vi "LSMcontroller_v66_improvedwfhandling.vi"() -> ()   [LabVIEW 2015] (continued)
                            n4742 = call "correctwaveformsizetemp.vi"("new sampling frequency (Hz)"=w1790, "start"=FALSE, "reference waveforms to"=w1802, "Analog waveforms in"=w1800, "stop"=FALSE, "Digital waveforms in"=w1807) -> ("analog wf out"=w1805:waveform(dbl)[], "Digital wf out"=w1803:digitalwaveform[], "measpoints"=w1792:i32)
                            n4743 = local read "wavdet"() -> (w1793:bool)
                            n4744 = local write "Analog Lines Plot"(w1805) -> ()
                            n4745 = call "GetNumCamFramesv2.vi"("Digital Waveform Graph"=w1803) -> ("Numeric"=w1804:i32)  [unwired: 10 in]
                            n4746 = local write "Digital Lines Plot"(w1803) -> ()
                            n4747 = call "waveformsAObuffer.vi"("AO wf in"=w1805, "command"="set") -> ()  [unwired: 1 out]
                            n4748 = call "waveformsDObuffer.vi"("DO wf in"=w1803, "command"="set") -> ()  [unwired: 1 out]
                            n4749 = local write "Total Camera Frames"(w1804) -> ()
                            n4750 = case shown="True" w1793 {
                              tunnel: w1792 -> [_ w1813]
                              frame False {
                              }
                              frame True {
                                n4751 = local write "# of frames"(w1813) -> ()
                              }
                            }
                          }
                        }
                      }
                    }
                  }
                  frame #5 {
                    w1815 = FALSE ("addAO")
                    n4752 = case shown="True" w1814 {
                      frame False {
                      }
                      frame True {
                        n4753 = local write "not loadedml"(FALSE ("not loadedml")) -> ()
                      }
                    }
                    n4754 = local read "finite samples"() -> (w1816:bool)
                    n4755 = local read "continuous"() -> (w1817:bool)
                    n4756 = local read "wavdet"() -> (w1818:bool)
                    n4757 = property on="Load Matlab Waveform" class="Bool (strict)"("Val(Sgnl)"=w1815) -> ()  [unwired: 2 in, 2 out]
                    n4758 = local write "changeAOmatlab"(w1815) -> ()
                    n4759 = call "2pparameters.vi"("command"="get") -> ("params out"=w1821:T10)  [unwired: 1 in]
                    n4760 = Bundle By Name(cluster=w1821, "finite"=w1816, "cont"=w1817, "wavdet"=w1818) -> (w1819:T10)
                    n4761 = call "2pparameters.vi"("Params in"=w1819, "command"="set") -> ()  [unwired: 1 out]
                  }
                }
              }
            }
          }
          event "Load Matlab Waveform DO": Value Change {
            n4762 = event-data() -> ("NewVal"=w1824:bool)  [unwired: 1 in, 5 out]
            n4763 = case shown="True" w1824 {
              frame False {
              }
              frame True {
                n4764 = stacked-sequence {
                  seq-local: [_ _ w1932 _ _] -> [_ _ _ w1947 _]
                  seq-local: [_ _ w1931 _ _] -> [_ _ _ w1946 _]
                  frame #0 {
                    n4765 = local read "Measurement"() -> (w1826:T4)
                    n4766 = case shown="\"X-Y-t movie\", Default" w1826 {
                      frame "X-Y-t movie", Default {
                        n4767 = local read "avpp"() -> (w1847:i32)
                        n4768 = local read "Angle ref"() -> (w1846:dbl)
                        n4769 = local read "ROI Type"() -> (w1845:u16)
                        n4770 = local read "xpixels ref"() -> (w1842:i32)
                        n4771 = local read "Vx-min ref"() -> (w1841:dbl)
                        n4772 = local read "Vx-max ref"() -> (w1840:dbl)
                        n4773 = local read "ypixels ref"() -> (w1838:i32)
                        n4774 = local read "Vy-min ref"() -> (w1839:dbl)
                        n4775 = local read "Vy-max ref"() -> (w1835:dbl)
                        n4776 = local read "Sampling rate"() -> (w1829:dbl)
                        n4777 = local read "finite samples"() -> (w1830:bool)
                        n4778 = local read "continuous"() -> (w1833:bool)
                        n4779 = local read "wavdet"() -> (w1834:bool)
                        n4780 = local read "# of frames"() -> (w1832:i32)
                        n4781 = local read "maxbufferAI"() -> (w1831:i32)
                        n4782 = local read "Override AI buffer"() -> (w1827:bool)
                        n4783 = call "2pparameters.vi"("command"="get") -> ("params out"=w1844:T10)  [unwired: 1 in]
                        n4784 = Bundle By Name(cluster=w1844, "type"="X-Y-t movie", "avpp"=w1847, "Angle Img"=w1846, "Xpixels Img"=w1842, "Vx-min Img"=w1841, "VX-max Img"=w1840, "Ypixels Img"=w1838, "Vy-min Img"=w1839, "Vy-max Img"=w1835, "srate"=w1829, "srate Img"=w1829, "finite"=w1830, "cont"=w1833, "wavdet"=w1834, "measpoints"=w1832, "maxbufferAI"=w1831, "Drawing Mode"=w1845, "Vz-reset"=0.0, "AIoverride"=w1827) -> (w1836:T10)
                        n4785 = call "2pparameters.vi"("Params in"=w1836, "command"="set") -> ()  [unwired: 1 out]
                      }
                      frame "X-Y-Z stack" {
                        n4786 = call "2pparameters.vi"("command"="get") -> ("params out"=w1851:T10)  [unwired: 1 in]
                        n4787 = Bundle By Name(cluster=w1851, "type"="X-Y-Z stack") -> (w1849:T10)
                        n4788 = call "2pparameters.vi"("Params in"=w1849, "command"="set") -> ()  [unwired: 1 out]
                      }
                      frame "Lifetime (scan)" {
                        n4789 = call "2pparameters.vi"("command"="get") -> ("params out"=w1856:T10)  [unwired: 1 in]
                        n4790 = Bundle By Name(cluster=w1856, "type"="Lifetime (scan)") -> (w1854:T10)
                        n4791 = call "2pparameters.vi"("Params in"=w1854, "command"="set") -> ()  [unwired: 1 out]
                      }
                      frame "Lifetime (contour)" {
                        n4792 = local read "Vy-min draw"() -> (w1866:dbl)
                        n4793 = local read "Vy-max draw"() -> (w1865:dbl)
                        n4794 = local read "Vx-min draw"() -> (w1868:dbl)
                        n4795 = local read "Vx-max draw"() -> (w1867:dbl)
                        n4796 = local read "xpixels ref"() -> (w1864:i32)
                        n4797 = local read "ypixels ref"() -> (w1863:i32)
                        n4798 = local read "ROI Type"() -> (w1862:u16)
                        n4799 = local read "srateAODOtt"() -> (w1873:dbl)
                        n4800 = local read "# of frames"() -> (w1878:i32)
                        n4801 = local read "refreshtime"() -> (w1870:dbl)
                        n4802 = local read "Pel"() -> (w1861:dbl)
                        n4803 = local read "bin"() -> (w1876:dbl)
                        n4804 = local read "Override AI buffer"() -> (w1859:bool)
                        n4805 = local read "finite samples"() -> (w1885:bool)
                        n4806 = local read "srateAODOtt"() -> (w1872:dbl)
                        n4807 = local read "srateAODOtt"() -> (w1879:dbl)
                        n4808 = local read "continuous"() -> (w1884:bool)
                        n4809 = local read "Angle ref"() -> (w1869:dbl)
                        n4810 = local read "wavdet"() -> (w1886:bool)
                        n4811 = local read "Vx-ref"() -> (w1881:dbl)
                        n4812 = local read "Vy-ref"() -> (w1883:dbl)
                        n4813 = local read "avpp"() -> (w1882:i32)
                        n4814 = call "tt_timeandsamples.vi"("bin"=w1876, "refreshtime"=w1870, "srateAODOtt"=w1873, "tot#ofsamples"=w1878) -> ("refreshrate"=w1874:dbl, "refreshbuffer"=w1875:i32, "timetracecycles"=w1880:i32)  [unwired: 5 in]
                        n4815 = local read "bin"() -> (w1877:dbl)
                        n4816 = call "2pparameters.vi"("command"="get") -> ("params out"=w1889:T10)  [unwired: 1 in]
                        n4817 = Bundle By Name(cluster=w1889, "Drawing Mode"=w1862, "measpoints"=w1878, "tt_cycles"=w1880, "refreshbuffer"=w1875, "refreshrate"=w1874, "Vx-ref"=w1881, "Vy-ref"=w1883, "srate"=w1872, "finite"=w1885, "cont"=w1884, "wavdet"=w1886, "avpp"=w1882, "srateAODO"=w1879, "bufferAI"=w1875, "bin"=w1877, "Angle Img"=w1869, "Vxminref"=w1868, "Vxmaxref"=w1867, "Vyminref"=w1866, "Vymaxref"=w1865, "Xpixels Img"=w1864, "Ypixels Img"=w1863, "Pel"=w1861, "Vz-reset"=0.0, "AIoverride"=w1859, "type"="Lifetime (contour)") -> (w1887:T10)
                        n4818 = Reciprocal(x=w1874) -> (1/x=w1871:dbl)
                        n4819 = local write "refreshtime"(w1871) -> ()
                        n4820 = call "2pparameters.vi"("Params in"=w1887, "command"="set") -> ()  [unwired: 1 out]
                      }
                      frame "X-Y-Z-t movie" {
                      }
                      frame "linescan" {
                      }
                      frame "Timetrace" {
                        n4821 = local read "Vy-min draw"() -> (w1899:dbl)
                        n4822 = local read "Vy-max draw"() -> (w1898:dbl)
                        n4823 = local read "Vx-min draw"() -> (w1901:dbl)
                        n4824 = local read "Vx-max draw"() -> (w1900:dbl)
                        n4825 = local read "xpixels ref"() -> (w1897:i32)
                        n4826 = local read "ypixels ref"() -> (w1896:i32)
                        n4827 = local read "ROI Type"() -> (w1895:u16)
                        n4828 = local read "srateAODOtt"() -> (w1906:dbl)
                        n4829 = local read "# of frames"() -> (w1911:i32)
                        n4830 = local read "refreshtime"() -> (w1903:dbl)
                        n4831 = local read "Pel"() -> (w1894:dbl)
                        n4832 = local read "bin"() -> (w1909:dbl)
                        n4833 = local read "Override AI buffer"() -> (w1892:bool)
                        n4834 = local read "finite samples"() -> (w1918:bool)
                        n4835 = local read "srateAODOtt"() -> (w1905:dbl)
                        n4836 = local read "srateAODOtt"() -> (w1912:dbl)
                        n4837 = local read "continuous"() -> (w1917:bool)
                        n4838 = local read "Angle ref"() -> (w1902:dbl)
                        n4839 = local read "wavdet"() -> (w1919:bool)
                        n4840 = local read "Vx-ref"() -> (w1914:dbl)
                        n4841 = local read "Vy-ref"() -> (w1916:dbl)
                        n4842 = local read "avpp"() -> (w1915:i32)
                        n4843 = call "tt_timeandsamples.vi"("bin"=w1909, "refreshtime"=w1903, "srateAODOtt"=w1906, "tot#ofsamples"=w1911) -> ("refreshrate"=w1907:dbl, "refreshbuffer"=w1908:i32, "timetracecycles"=w1913:i32)  [unwired: 5 in]
                        n4844 = local read "bin"() -> (w1910:dbl)
                        n4845 = call "2pparameters.vi"("command"="get") -> ("params out"=w1922:T10)  [unwired: 1 in]
                        n4846 = Bundle By Name(cluster=w1922, "Drawing Mode"=w1895, "measpoints"=w1911, "tt_cycles"=w1913, "refreshbuffer"=w1908, "refreshrate"=w1907, "Vx-ref"=w1914, "Vy-ref"=w1916, "srate"=w1905, "finite"=w1918, "cont"=w1917, "wavdet"=w1919, "avpp"=w1915, "srateAODO"=w1912, "bufferAI"=w1908, "bin"=w1910, "Angle Img"=w1902, "Vxminref"=w1901, "Vxmaxref"=w1900, "Vyminref"=w1899, "Vymaxref"=w1898, "Xpixels Img"=w1897, "Ypixels Img"=w1896, "Pel"=w1894, "Vz-reset"=0.0, "AIoverride"=w1892, "type"="Timetrace") -> (w1920:T10)
                        n4847 = Reciprocal(x=w1907) -> (1/x=w1904:dbl)
                        n4848 = local write "refreshtime"(w1904) -> ()
                        n4849 = call "2pparameters.vi"("Params in"=w1920, "command"="set") -> ()  [unwired: 1 out]
                      }
                      frame "Lifetime (point)" {
                      }
                    }
                    n4850 = local write "changeDOmatlab"(TRUE ("addAO")) -> ()
                  }
                  frame #1 {
                    w1925 = FALSE ("wavdet")
                    n4851 = call "2pparameters.vi"("command"="get") -> ("params out"=w1929:T10)  [unwired: 1 in]
                    n4852 = Bundle By Name(cluster=w1929, "finite"=w1925, "cont"=w1925, "wavdet"=TRUE) -> (w1926:T10)
                    n4853 = call "2pparameters.vi"("Params in"=w1926, "command"="set") -> ()  [unwired: 1 out]
                  }
                  frame #2 {
                    n4854 = local read "DO channels"() -> (w1934:u16)
                    n4855 = call "2pparameters.vi"("command"="get") -> ("params out"=w1936:T10)  [unwired: 1 in]
                    n4856 = Unbundle By Name(w1936) -> ("aDO"=w1935:u32[])
                    n4857 = Search 1D Array(1D array=w1935, element=w1934) -> (index of element=w1932:i32)  [unwired: 1 in]
                    n4858 = Greater?(x=w1932, y=-1) -> (0:w1931:bool)
                    n4859 = case shown="True" w1931 {
                      tunnel: w1932 -> [_ w1943]
                      frame False {
                      }
                      frame True {
                        n4860 = local read "Meastab"() -> (w1939:enum32{"X-Y Image", "Linescan", "Timetrace"})
                        n4861 = local read "Matlab waveform path DO"() -> (w1941:path)
                        n4862 = local read "Matlab padding value DO"() -> (w1942:dbl)
                        n4863 = case shown="\"Timetrace\"" w1939 {
                          tunnel: [w1944 w1945] -> w1938
                          frame "X-Y Image", Default {
                            n4864 = local read "Sampling rate"() -> (w1944:dbl)
                          }
                          frame "Timetrace" {
                            n4865 = local read "srateAODOtt"() -> (w1945:dbl)
                          }
                        }
                        n4866 = call "matlabwfexistsdialogue.vi"("Matlab waveform path"=w1941) -> ("mtalab waveform path out"=w1940:path)
                        n4867 = call "replace DO matlab param.vi"("Sampling frequency (Hz)"=w1938, "matlab wave number"=w1940, "index of DO wave"=w1943, "padding value"=w1942) -> ()  [unwired: 7 in]
                      }
                    }
                  }
                  frame #3 {
                    n4868 = case shown="True" w1946 {
                      tunnel: w1947 -> [_ w1956]
                      frame False {
                      }
                      frame True {
                        n4869 = local read "Meastab"() -> (w1951:enum32{"X-Y Image", "Linescan", "Timetrace"})
                        n4870 = call "waveformparamsv2.vi"("command"="get") -> ("Params out"=w1969:T14)  [unwired: 4 in, 2 out]
                        n4871 = Unbundle By Name(w1969) -> ("DO parameters"=w1968:T17)
                        n4872 = case shown="\"Timetrace\"" w1951 {
                          tunnel: [w1971 w1972] -> w1950
                          frame "X-Y Image", Default {
                            n4873 = local read "Sampling rate"() -> (w1971:dbl)
                          }
                          frame "Timetrace" {
                            n4874 = local read "srateAODOtt"() -> (w1972:dbl)
                          }
                        }
                        n4875 = Index Array(array=w1968, index=w1956) -> (element=w1955:T18)
                        n4876 = call "waveformsDObuffer.vi"("command"="get") -> ("DO wf out"=w1966:digitalwaveform[])  [unwired: 1 in]
                        n4877 = property on="refwf" class="Ring (strict)"() -> ("RingText.Text"=w1958:string)  [unwired: 2 in, 2 out]
                        n4878 = call "matlabDOwffromparam.vi"("waveform params"=w1955) -> ("digital waveform"=w1954:digitalwaveform)
                        n4879 = Replace Array Subset(array=w1966, new element=w1954, index=w1956) -> (w1957:digitalwaveform[])
                        n4880 = call "waveformsAObuffer.vi"("command"="get") -> ("AO wf out"=w1965:waveform(dbl)[])  [unwired: 1 in]
                        n4881 = local read "wavdet"() -> (w1953:bool)
                        n4882 = call "correctwaveformsizetemp.vi"("new sampling frequency (Hz)"=w1950, "start"=FALSE, "reference waveforms to"=w1958, "Analog waveforms in"=w1965, "stop"=FALSE, "Digital waveforms in"=w1957) -> ("analog wf out"=w1961:waveform(dbl)[], "Digital wf out"=w1959:digitalwaveform[], "measpoints"=w1952:i32)
                        n4883 = local write "Analog Lines Plot"(w1961) -> ()
                        n4884 = call "GetNumCamFramesv2.vi"("Digital Waveform Graph"=w1959) -> ("Numeric"=w1960:i32)  [unwired: 10 in]
                        n4885 = local write "Digital Lines Plot"(w1959) -> ()
                        n4886 = case shown="True" w1953 {
                          tunnel: w1952 -> [_ w1973]
                          frame False {
                          }
                          frame True {
                            n4887 = local write "# of frames"(w1973) -> ()
                          }
                        }
                        n4888 = call "waveformsAObuffer.vi"("AO wf in"=w1961, "command"="set") -> ()  [unwired: 1 out]
                        n4889 = call "waveformsDObuffer.vi"("DO wf in"=w1959, "command"="set") -> ()  [unwired: 1 out]
                        n4890 = local write "Total Camera Frames"(w1960) -> ()
                      }
                    }
                  }
                  frame #4 {
                    w1975 = FALSE ("addAO")
                    n4891 = local read "finite samples"() -> (w1976:bool)
                    n4892 = local read "continuous"() -> (w1977:bool)
                    n4893 = local read "wavdet"() -> (w1978:bool)
                    n4894 = call "2pparameters.vi"("command"="get") -> ("params out"=w1981:T10)  [unwired: 1 in]
                    n4895 = Bundle By Name(cluster=w1981, "finite"=w1976, "cont"=w1977, "wavdet"=w1978) -> (w1979:T10)
                    n4896 = local write "not loadedDOml"(FALSE ("not loadedDO")) -> ()
                    n4897 = local write "changeDOmatlab"(w1975) -> ()
                    n4898 = property on="Load Matlab Waveform DO" class="Bool (strict)"("Val(Sgnl)"=w1975) -> ()  [unwired: 2 in, 2 out]
                    n4899 = call "2pparameters.vi"("Params in"=w1979, "command"="set") -> ()  [unwired: 1 out]
                  }
                }
              }
            }
          }
          event "Add settings": Value Change {
            n4900 = event-data() -> ("NewVal"=w1983:bool)  [unwired: 1 in, 5 out]
            n4901 = case shown="True" w1983 {
              frame False {
              }
              frame True {
                n4902 = stacked-sequence {
                  frame #0 {
                    n4903 = call "wfsettings.vi"("command"="get") -> ("wfsettings out"=w1986:T27)  [unwired: 2 in, 1 out]
                    n4904 = in-place {
                      n4905 = in-place-cluster #53(w1986) -> ("settings names"=w1991:string[], "settings locations"=w1993:path[])
                      n4906 = local read "Setting location"() -> (w1989:path)
                      n4907 = local read "Nickname"() -> (w1988:string)
                      n4908 = Build Array (concatenate)(w1991, w1988) -> (w1990:string[])
                      n4909 = property on="Loaded settings" class="Ring (strict)"("Strings []"=w1990) -> ()  [unwired: 2 in, 2 out]
                      n4910 = Build Array (concatenate)(w1993, w1989) -> (w1992:path[])
                      n4911 = in-place-cluster #53("settings names"=w1990, "settings locations"=w1992) -> (w1984:T27)
                    }
                    n4912 = call "wfsettings.vi"("wfsettings in"=w1984, "command"="set") -> ()  [unwired: 1 in, 2 out]
                  }
                  frame #1 {
                    n4913 = property on="Add settings" class="Bool (strict)"("Val(Sgnl)"=FALSE ("Value (Signaling)")) -> ()  [unwired: 2 in, 2 out]
                  }
                }
              }
            }
          }
          event "Rem setting": Value Change {
            n4914 = event-data() -> ("NewVal"=w1995:bool)  [unwired: 1 in, 5 out]
            n4915 = case shown="True" w1995 {
              frame False {
              }
              frame True {
                n4916 = stacked-sequence {
                  frame #0 {
                    n4917 = call "wfsettings.vi"("command"="get") -> ("wfsettings out"=w1998:T27)  [unwired: 2 in, 1 out]
                    n4918 = in-place {
                      n4919 = in-place-cluster #54(w1998) -> ("settings names"=w2003:string[], "settings locations"=w2001:path[])
                      n4920 = property on="Loaded settings" class="Ring (strict)"() -> ("RingText.Text"=w2004:string)  [unwired: 2 in, 2 out]
                      n4921 = Search 1D Array(1D array=w2003, element=w2004) -> (index of element=w2005:i32)  [unwired: 1 in]
                      n4922 = Delete From Array(array=w2003, index=w2005) -> (array with subset deleted=w2002:string[])  [unwired: 1 in, 1 out]
                      n4923 = Delete From Array(array=w2001, index=w2005) -> (array with subset deleted=w2000:path[])  [unwired: 1 in, 1 out]
                      n4924 = property on="Loaded settings" class="Ring (strict)"("Strings []"=w2002) -> ()  [unwired: 2 in, 2 out]
                      n4925 = in-place-cluster #54("settings names"=w2002, "settings locations"=w2000) -> (w1996:T27)
                    }
                    n4926 = call "wfsettings.vi"("wfsettings in"=w1996, "command"="set") -> ()  [unwired: 1 in, 2 out]
                  }
                  frame #1 {
                    n4927 = property on="Rem setting" class="Bool (strict)"("Val(Sgnl)"=FALSE ("Value (Signaling)")) -> ()  [unwired: 2 in, 2 out]
                  }
                }
              }
            }
          }
          event "Update settings": Value Change {
            n4928 = event-data() -> ("NewVal"=w2007:bool)  [unwired: 1 in, 5 out]
            n4929 = case shown="True" w2007 {
              frame False {
              }
              frame True {
                n4930 = stacked-sequence {
                  frame #0 {
                    n4931 = local read "Measurement"() -> (w2008:T4)
                    n4932 = case shown="\"Timetrace\"" w2008 {
                      frame "X-Y-t movie", Default {
                        n4933 = local read "avpp"() -> (w2029:i32)
                        n4934 = local read "Angle ref"() -> (w2028:dbl)
                        n4935 = local read "ROI Type"() -> (w2027:u16)
                        n4936 = local read "xpixels ref"() -> (w2024:i32)
                        n4937 = local read "Vx-min ref"() -> (w2023:dbl)
                        n4938 = local read "Vx-max ref"() -> (w2022:dbl)
                        n4939 = local read "ypixels ref"() -> (w2020:i32)
                        n4940 = local read "Vy-min ref"() -> (w2021:dbl)
                        n4941 = local read "Vy-max ref"() -> (w2017:dbl)
                        n4942 = local read "Sampling rate"() -> (w2011:dbl)
                        n4943 = local read "finite samples"() -> (w2012:bool)
                        n4944 = local read "continuous"() -> (w2015:bool)
                        n4945 = local read "wavdet"() -> (w2016:bool)
                        n4946 = local read "# of frames"() -> (w2014:i32)
                        n4947 = local read "maxbufferAI"() -> (w2013:i32)
                        n4948 = local read "Override AI buffer"() -> (w2009:bool)
                        n4949 = call "2pparameters.vi"("command"="get") -> ("params out"=w2026:T10)  [unwired: 1 in]
                        n4950 = Bundle By Name(cluster=w2026, "type"="X-Y-t movie", "avpp"=w2029, "Angle Img"=w2028, "Xpixels Img"=w2024, "Vx-min Img"=w2023, "VX-max Img"=w2022, "Ypixels Img"=w2020, "Vy-min Img"=w2021, "Vy-max Img"=w2017, "srate"=w2011, "srate Img"=w2011, "finite"=w2012, "cont"=w2015, "wavdet"=w2016, "measpoints"=w2014, "maxbufferAI"=w2013, "Drawing Mode"=w2027, "Vz-reset"=0.0, "AIoverride"=w2009) -> (w2018:T10)
                        n4951 = call "2pparameters.vi"("Params in"=w2018, "command"="set") -> ()  [unwired: 1 out]
                      }
                      frame "X-Y-Z stack" {
                        n4952 = call "2pparameters.vi"("command"="get") -> ("params out"=w2033:T10)  [unwired: 1 in]
                        n4953 = Bundle By Name(cluster=w2033, "type"="X-Y-Z stack") -> (w2031:T10)
                        n4954 = call "2pparameters.vi"("Params in"=w2031, "command"="set") -> ()  [unwired: 1 out]
                      }
                      frame "Lifetime (scan)" {
                        n4955 = call "2pparameters.vi"("command"="get") -> ("params out"=w2038:T10)  [unwired: 1 in]
                        n4956 = Bundle By Name(cluster=w2038, "type"="Lifetime (scan)") -> (w2036:T10)
                        n4957 = call "2pparameters.vi"("Params in"=w2036, "command"="set") -> ()  [unwired: 1 out]
                      }
                      frame "Lifetime (contour)" {
                        n4958 = local read "Vy-min draw"() -> (w2048:dbl)
                        n4959 = local read "Vy-max draw"() -> (w2047:dbl)
                        n4960 = local read "Vx-min draw"() -> (w2050:dbl)
                        n4961 = local read "Vx-max draw"() -> (w2049:dbl)
                        n4962 = local read "xpixels ref"() -> (w2046:i32)
                        n4963 = local read "ypixels ref"() -> (w2045:i32)
                        n4964 = local read "ROI Type"() -> (w2044:u16)
                        n4965 = local read "srateAODOtt"() -> (w2055:dbl)
                        n4966 = local read "# of frames"() -> (w2060:i32)
                        n4967 = local read "refreshtime"() -> (w2052:dbl)
                        n4968 = local read "Pel"() -> (w2043:dbl)
                        n4969 = local read "bin"() -> (w2058:dbl)
                        n4970 = local read "Override AI buffer"() -> (w2041:bool)
                        n4971 = local read "finite samples"() -> (w2067:bool)
                        n4972 = local read "srateAODOtt"() -> (w2054:dbl)
                        n4973 = local read "srateAODOtt"() -> (w2061:dbl)
                        n4974 = local read "continuous"() -> (w2066:bool)
                        n4975 = local read "Angle ref"() -> (w2051:dbl)
                        n4976 = local read "wavdet"() -> (w2068:bool)
                        n4977 = local read "Vx-ref"() -> (w2063:dbl)
                        n4978 = local read "Vy-ref"() -> (w2065:dbl)
                        n4979 = local read "avpp"() -> (w2064:i32)
                        n4980 = call "tt_timeandsamples.vi"("bin"=w2058, "refreshtime"=w2052, "srateAODOtt"=w2055, "tot#ofsamples"=w2060) -> ("refreshrate"=w2056:dbl, "refreshbuffer"=w2057:i32, "timetracecycles"=w2062:i32)  [unwired: 5 in]
                        n4981 = local read "bin"() -> (w2059:dbl)
                        n4982 = call "2pparameters.vi"("command"="get") -> ("params out"=w2071:T10)  [unwired: 1 in]
                        n4983 = Bundle By Name(cluster=w2071, "Drawing Mode"=w2044, "measpoints"=w2060, "tt_cycles"=w2062, "refreshbuffer"=w2057, "refreshrate"=w2056, "Vx-ref"=w2063, "Vy-ref"=w2065, "srate"=w2054, "finite"=w2067, "cont"=w2066, "wavdet"=w2068, "avpp"=w2064, "srateAODO"=w2061, "bufferAI"=w2057, "bin"=w2059, "Angle Img"=w2051, "Vxminref"=w2050, "Vxmaxref"=w2049, "Vyminref"=w2048, "Vymaxref"=w2047, "Xpixels Img"=w2046, "Ypixels Img"=w2045, "Pel"=w2043, "Vz-reset"=0.0, "AIoverride"=w2041, "type"="Lifetime (contour)") -> (w2069:T10)
                        n4984 = Reciprocal(x=w2056) -> (1/x=w2053:dbl)
                        n4985 = local write "refreshtime"(w2053) -> ()
                        n4986 = call "2pparameters.vi"("Params in"=w2069, "command"="set") -> ()  [unwired: 1 out]
                      }
                      frame "X-Y-Z-t movie" {
                      }
                      frame "linescan" {
                      }
                      frame "Timetrace" {
                        n4987 = local read "Vy-min draw"() -> (w2081:dbl)
                        n4988 = local read "Vy-max draw"() -> (w2080:dbl)
                        n4989 = local read "Vx-min draw"() -> (w2083:dbl)
                        n4990 = local read "Vx-max draw"() -> (w2082:dbl)
                        n4991 = local read "xpixels ref"() -> (w2079:i32)
                        n4992 = local read "ypixels ref"() -> (w2078:i32)
                        n4993 = local read "ROI Type"() -> (w2077:u16)
                        n4994 = local read "srateAODOtt"() -> (w2088:dbl)
                        n4995 = local read "# of frames"() -> (w2093:i32)
                        n4996 = local read "refreshtime"() -> (w2085:dbl)
                        n4997 = local read "Pel"() -> (w2076:dbl)
                        n4998 = local read "bin"() -> (w2091:dbl)
                        n4999 = local read "Override AI buffer"() -> (w2074:bool)
                        n5000 = local read "finite samples"() -> (w2100:bool)
                        n5001 = local read "srateAODOtt"() -> (w2087:dbl)
                        n5002 = local read "srateAODOtt"() -> (w2094:dbl)
                        n5003 = local read "continuous"() -> (w2099:bool)
                        n5004 = local read "Angle ref"() -> (w2084:dbl)
                        n5005 = local read "wavdet"() -> (w2101:bool)
                        n5006 = local read "Vx-ref"() -> (w2096:dbl)
                        n5007 = local read "Vy-ref"() -> (w2098:dbl)
                        n5008 = local read "avpp"() -> (w2097:i32)
                        n5009 = call "tt_timeandsamples.vi"("bin"=w2091, "refreshtime"=w2085, "srateAODOtt"=w2088, "tot#ofsamples"=w2093) -> ("refreshrate"=w2089:dbl, "refreshbuffer"=w2090:i32, "timetracecycles"=w2095:i32)  [unwired: 5 in]
                        n5010 = local read "bin"() -> (w2092:dbl)
                        n5011 = call "2pparameters.vi"("command"="get") -> ("params out"=w2104:T10)  [unwired: 1 in]
                        n5012 = Bundle By Name(cluster=w2104, "Drawing Mode"=w2077, "measpoints"=w2093, "tt_cycles"=w2095, "refreshbuffer"=w2090, "refreshrate"=w2089, "Vx-ref"=w2096, "Vy-ref"=w2098, "srate"=w2087, "finite"=w2100, "cont"=w2099, "wavdet"=w2101, "avpp"=w2097, "srateAODO"=w2094, "bufferAI"=w2090, "bin"=w2092, "Angle Img"=w2084, "Vxminref"=w2083, "Vxmaxref"=w2082, "Vyminref"=w2081, "Vymaxref"=w2080, "Xpixels Img"=w2079, "Ypixels Img"=w2078, "Pel"=w2076, "Vz-reset"=0.0, "AIoverride"=w2074, "type"="Timetrace") -> (w2102:T10)
                        n5013 = Reciprocal(x=w2089) -> (1/x=w2086:dbl)
                        n5014 = local write "refreshtime"(w2086) -> ()
                        n5015 = call "2pparameters.vi"("Params in"=w2102, "command"="set") -> ()  [unwired: 1 out]
                      }
                      frame "Lifetime (point)" {
                      }
                    }
                  }
                  frame #1 {
                    w2107 = FALSE ("wavdet")
                    n5016 = call "2pparameters.vi"("command"="get") -> ("params out"=w2111:T10)  [unwired: 1 in]
                    n5017 = Bundle By Name(cluster=w2111, "finite"=w2107, "cont"=w2107, "wavdet"=TRUE) -> (w2108:T10)
                    n5018 = call "2pparameters.vi"("Params in"=w2108, "command"="set") -> ()  [unwired: 1 out]
                  }
                  frame #2 {
                    n5019 = property on="Loaded settings" class="Ring (strict)"() -> ("RingText.Text"=w2113:string)  [unwired: 2 in, 2 out]
                    n5020 = control-ref of="Analog Lines Plot"() -> (w2115:refnum<vi>)
                    n5021 = control-ref of="Digital Lines Plot"() -> (w2114:refnum<vi>)
                    n5022 = call "Usedlinesfromsettingsfile.vi"("sertting"=w2113) -> ("used AO names"=w2119:string[], "used AO lines"=w2118:tag[], "used DO names"=w2117:string[], "used DO lines"=w2116:tag[])
                    n5023 = call "loadAODOwfparamsfromsettingsfile.vi"("sertting"=w2113) -> ()
                    n5024 = call "prepAOWaveplot.vi"("WaveformGraph in"=w2115, "Analog Used Names"=w2119) -> ()  [unwired: 1 in]
                    n5025 = local write "Analog Used Names"(w2119) -> ()
                    n5026 = local write "Analog Used Lines"(w2118) -> ()
                    n5027 = call "prepDOWaveplot.vi"("DigitalGraph in"=w2114, "used DO names"=w2117) -> ()  [unwired: 1 in]
                    n5028 = local write "Digital Used Names"(w2117) -> ()
                    n5029 = local write "Digital Used Lines"(w2116) -> ()
                  }
                  frame #3 {
                    n5030 = call "waveformparamsv2.vi"("command"="get") -> ("Params out"=w2136:T14)  [unwired: 4 in, 2 out]
                    n5031 = Unbundle By Name(w2136) -> ("AO parameters"=w2137:T15, "DO parameters"=w2138:T17)
                    n5032 = for {
                      tunnel: w2137 -> [w2158] mode=indexing
                      tunnel: [w2156] -> w2139 mode=indexing
                      tunnel: [w2155] -> w2124 mode=indexing
                      tunnel: [w2153] -> w2127 mode=indexing
                      i -> [w2157]
                      n5033 = Unbundle By Name(w2158) -> ("AOtab"=w2159:dbl)
                      n5034 = To Long Integer(number=w2159) -> (32bit integer=w2152:i32)
                      n5035 = case shown="2" w2152 {
                        tunnel: w2158 -> [_ w2170 w2172 w2174]
                        tunnel: [_ w2169 w2171 w2173] -> w2154
                        frame -1 {
                        }
                        frame 0, Default {
                          n5036 = call "generateRampedSquareWave_fromAOparameters.vi"("AO params"=w2170) -> ("Waveform"=w2169:waveform(dbl))  [unwired: 1 out]
                        }
                        frame 1 {
                          n5037 = call "generateTriWave_fromAOparameters.vi"("AO params"=w2172) -> ("Waveform"=w2171:waveform(dbl))  [unwired: 1 out]
                        }
                        frame 2 {
                          n5038 = call "matlabAOwffromparam.vi"("Cluster"=w2174) -> ("Waveform"=w2173:waveform(dbl))  [unwired: 1 out]
                        }
                      }
                      n5039 = case shown="0" w2157 {
                        tunnel: [w2164 -1] -> w2156
                        tunnel: [w2163 w2167] -> w2155
                        tunnel: w2154 -> [w2163 w2167]
                        tunnel: [w2160 -1.0] -> w2153
                        frame 0 {
                          n5040 = Unbundle By Name(w2163) -> ("dt"=w2162:dbl, "Y"=w2165:dbl[])
                          n5041 = Reciprocal(x=w2162) -> (1/x=w2161:dbl)
                          n5042 = Array Size(array=w2165) -> (size(s)=w2164:i32)
                          n5043 = Round To Nearest(number=w2161) -> (nearest integer value=w2160:dbl)
                        }
                        frame 1, Default {
                        }
                      }
                    }
                    n5044 = Index Array(array=w2139, index=0) -> (element=w2141:i32)
                    n5045 = Index Array(array=w2127, index=0) -> (element=w2126:dbl)
                    n5046 = for {
                      tunnel: w2138 -> [w2146] mode=indexing
                      tunnel: [w2144] -> w2125 mode=indexing
                      tunnel: w2141 -> [w2143]
                      n5047 = Unbundle By Name(w2146) -> ("DOtab"=w2145:dbl)
                      n5048 = case shown="0, Default" w2145 {
                        tunnel: w2146 -> [w2149 w2151]
                        tunnel: w2143 -> [w2148 _]
                        tunnel: [w2147 w2150] -> w2144
                        frame 0, Default {
                          n5049 = call "simple digital from wf params.vi"("waveform params"=w2149, "number of samples"=w2148) -> ("digital waveform"=w2147:digitalwaveform)
                        }
                        frame 1 {
                          n5050 = call "matlabDOwffromparam.vi"("waveform params"=w2151) -> ("digital waveform"=w2150:digitalwaveform)
                        }
                      }
                    }
                    n5051 = property on="refwf" class="Ring (strict)"() -> ("RingText.Text"=w2129:string)  [unwired: 2 in, 2 out]
                    n5052 = call "correctwaveformsizetemp.vi"("new sampling frequency (Hz)"=w2126, "start"=FALSE, "reference waveforms to"=w2129, "Analog waveforms in"=w2124, "stop"=FALSE, "Digital waveforms in"=w2125) -> ("analog wf out"=w2123:waveform(dbl)[], "Digital wf out"=w2122:digitalwaveform[], "measpoints"=w2120:i32)
                    n5053 = local read "wavdet"() -> (w2121:bool)
                    n5054 = case shown="True" w2121 {
                      tunnel: w2120 -> [_ w2142]
                      frame False {
                      }
                      frame True {
                        n5055 = local write "# of frames"(w2142) -> ()
                      }
                    }
                    n5056 = local write "Analog Lines Plot"(w2123) -> ()
                    n5057 = local write "Digital Lines Plot"(w2122) -> ()
                    n5058 = call "GetNumCamFramesv2.vi"("Digital Waveform Graph"=w2122) -> ("Numeric"=w2134:i32)  [unwired: 10 in]
                    n5059 = call "waveformsAObuffer.vi"("AO wf in"=w2123, "command"="set") -> ()  [unwired: 1 out]
                    n5060 = call "waveformsDObuffer.vi"("DO wf in"=w2122, "command"="set") -> ()  [unwired: 1 out]
                    n5061 = local write "Total Camera Frames"(w2134) -> ()
                  }
                  frame #4 {
                    n5062 = local read "AO channels"() -> (w2175:u32)
                    n5063 = call "2pparameters.vi"("command"="get") -> ("params out"=w2177:T10)  [unwired: 1 in]
                    n5064 = Unbundle By Name(w2177) -> ("aAO"=w2176:u32[])
                    n5065 = Search 1D Array(1D array=w2176, element=w2175) -> (index of element=w2179:i32)  [unwired: 1 in]
                    n5066 = Equal?(x=w2179, y=-1.0) -> (x = y?=w2180:bool)
                    n5067 = case shown="False" w2180 {
                      tunnel: w2179 -> [w2205 _]
                      frame False {
                        n5068 = call "waveformparamsv2.vi"("command"="get") -> ("Params out"=w2188:T14)  [unwired: 4 in, 2 out]
                        n5069 = Unbundle By Name(w2188) -> ("AO parameters"=w2187:T15)
                        n5070 = Index Array(array=w2187, index=w2205) -> (element=w2204:T16)
                        n5071 = Unbundle By Name(w2204) -> ("AOtab"=w2185:dbl, "Repeats"=w2203:dbl, "Cycles"=w2202:dbl, "Start amplitude (V)"=w2201:dbl, "Baseline (V)"=w2200:dbl, "Step size (V)"=w2199:dbl, "DC (%)"=w2198:dbl, "Sampling frequency (Hz)"=w2197:dbl, "Period (ms)"=w2196:dbl, "Offset (V)"=w2195:dbl, "Amplitude (V)"=w2194:dbl, "Frequency"=w2193:dbl, "Tri Repeats"=w2192:dbl, "phase shift (ms)"=w2191:dbl, "Pulses"=w2190:dbl, "Tri phase"=w2186:dbl, "padding value"=w2182:dbl, "Matlab wave file"=w2183:path)
                        n5072 = To Unsigned Long Integer(number=w2185) -> (unsigned 32bit integer=w2184:u32)
                        n5073 = local write "Build analog waveform tabs"(w2184) -> ()
                        n5074 = local write "Matlab waveform path"(w2183) -> ()
                        n5075 = local write "phase shift (ms)"(w2191) -> ()
                        n5076 = local write "Repeats"(w2203) -> ()
                        n5077 = local write "Cycles"(w2202) -> ()
                        n5078 = local write "Amplitude (V)"(w2194) -> ()
                        n5079 = local write "Matlab padding value"(w2182) -> ()
                        n5080 = local write "Tri padding value"(w2182) -> ()
                        n5081 = local write "Start amplitude (V)"(w2201) -> ()
                        n5082 = local write "Tri Phase (s)"(w2186) -> ()
                        n5083 = local write "Period (ms)"(w2196) -> ()
                        n5084 = local write "Tri Repeats"(w2192) -> ()
                        n5085 = local write "Offset (V)"(w2195) -> ()
                        n5086 = local write "Frequency"(w2193) -> ()
                        n5087 = local write "Pulses"(w2190) -> ()
                        n5088 = local write "padding value"(w2182) -> ()
                        n5089 = local write "Sampling rate \ncurrent wf"(w2197) -> ()
                        n5090 = local write "Baseline (V)"(w2200) -> ()
                        n5091 = local write "Step size (V)"(w2199) -> ()
                        n5092 = local write "DC (%)"(w2198) -> ()
                      }
                      frame True {
                      }
                    }
                  }
                  frame #5 {
                    n5093 = local read "DO channels"() -> (w2208:u16)
                    n5094 = call "2pparameters.vi"("command"="get") -> ("params out"=w2210:T10)  [unwired: 1 in]
                    n5095 = Unbundle By Name(w2210) -> ("aDO"=w2209:u32[])
                    n5096 = Search 1D Array(1D array=w2209, element=w2208) -> (index of element=w2207:i32)  [unwired: 1 in]
                    n5097 = Equal?(x=w2207, y=-1.0) -> (x = y?=w2206:bool)
                    n5098 = case shown="False" w2206 {
                      tunnel: w2207 -> [w2225 _]
                      frame False {
                        n5099 = call "waveformparamsv2.vi"("command"="get") -> ("Params out"=w2219:T14)  [unwired: 4 in, 2 out]
                        n5100 = Unbundle By Name(w2219) -> ("DO parameters"=w2217:T17)
                        n5101 = Index Array(array=w2217, index=w2225) -> (element=w2224:T18)
                        n5102 = Unbundle By Name(w2224) -> ("Digital DC (%)"=w2223:dbl, "Digital phase"=w2222:dbl, "Digital Freq (Hz)"=w2221:dbl, "Sampling frequency (Hz)"=w2220:dbl, "Digital time offset (s)"=w2216:dbl, "padding value"=w2215:dbl, "matlab wave file"=w2214:path, "DOtab"=w2213:dbl)
                        n5103 = local write "Build digital waveform tabs"(w2213) -> ()
                        n5104 = local write "Digital DC (%)"(w2223) -> ()
                        n5105 = local write "Matlab waveform path DO"(w2214) -> ()
                        n5106 = local write "Sampling rate \ncurrent wf"(w2220) -> ()
                        n5107 = local write "Digital time offset (s)"(w2216) -> ()
                        n5108 = local write "Matlab padding value DO"(w2215) -> ()
                        n5109 = local write "Digital padding value"(w2215) -> ()
                        n5110 = local write "Digital Freq (Hz)"(w2221) -> ()
                        n5111 = local write "Digital phase (s)"(w2222) -> ()
                      }
                      frame True {
                      }
                    }
                  }
                  frame #6 {
                    n5112 = local read "finite samples"() -> (w2227:bool)
                    n5113 = local read "continuous"() -> (w2228:bool)
                    n5114 = local read "wavdet"() -> (w2229:bool)
                    n5115 = call "2pparameters.vi"("command"="get") -> ("params out"=w2232:T10)  [unwired: 1 in]
                    n5116 = Bundle By Name(cluster=w2232, "finite"=w2227, "cont"=w2228, "wavdet"=w2229) -> (w2230:T10)
                    n5117 = property on="Update settings" class="Bool (strict)"("Val(Sgnl)"=FALSE ("Value (Signaling)")) -> ()  [unwired: 2 in, 2 out]
                    n5118 = call "2pparameters.vi"("Params in"=w2230, "command"="set") -> ()  [unwired: 1 out]
                  }
                }
              }
            }
          }
          event "Digital phase (s)", "Digital DC (%)", "Digital Freq (Hz)", "Digital padding value", "Digital time offset (s)": Value Change {
            n5119 = event-data() -> ()  [unwired: 1 in, 6 out]
            n5120 = local write "not loadedDO"(TRUE ("not loadedDO")) -> ()
          }
          event "Matlab padding value DO", "Matlab waveform path DO": Value Change {
            n5121 = event-data() -> ()  [unwired: 1 in, 6 out]
            n5122 = local write "not loadedDOml"(TRUE ("not loadedDO")) -> ()
          }
          event "phase shift (ms)", "Pulses", "Baseline (V)", "Step size (V)", "Start amplitude (V)", "Period (ms)", "DC (%)", "Cycles", "Repeats", "padding value": Value Change {
            n5123 = event-data() -> ()  [unwired: 1 in, 6 out]
            n5124 = local write "not loaded"(TRUE ("not loaded")) -> ()
          }
          event "Tri Repeats", "Amplitude (V)", "Offset (V)", "Frequency", "Tri Phase (s)", "Tri padding value": Value Change {
            n5125 = event-data() -> ()  [unwired: 1 in, 6 out]
            n5126 = local write "not loadedtri"(TRUE ("not loadedtri")) -> ()
          }
          event "Matlab waveform path", "Matlab padding value": Value Change {
            n5127 = event-data() -> ()  [unwired: 1 in, 6 out]
            n5128 = local write "not loadedml"(TRUE ("not loadedml")) -> ()
          }
          event "Exit": Value Change {
            n5129 = event-data() -> ("NewVal"=w2239:bool)  [unwired: 1 in]
          }
        }
        n5130 = Wait (ms)(milliseconds to wait=u32 50) -> ()  [unwired: 1 out]
      }
    }
    frame #3 {
      w6663 = FALSE ("Value (Signaling)")
      n5131 = property on="Start" class="Bool (strict)"("Val(Sgnl)"=w6663) -> ()  [unwired: 2 in, 2 out]
      n5132 = property on="Exit" class="Bool (strict)"("Val(Sgnl)"=w6663) -> ()  [unwired: 2 in, 2 out]
      n5133 = property on="Stop" class="Bool (strict)"("Val(Sgnl)"=w6663) -> ()  [unwired: 2 in, 2 out]
      n5134 = flat-sequence {
        frame #0 {
          w6664 = u16 1 items=["OD 0"=1, "OD 0.5"=2, "OD 1"=3, "OD 2"=4, "OD 3"=5, "OD 4"=6] ("New ODfilt")
          n5135 = local read "ODfilt"() -> (w6665:u16)
          n5136 = call "filterwheelcontrol_nothorlabslib.vi"("Current OD filt"=w6665, "New ODfilt"=w6664) -> ()  [unwired: 1 in]
        }
        frame #1 {
          n5137 = Wait (ms)(milliseconds to wait=u32 1000) -> ()  [unwired: 1 out]
        }
      }
    }
  }
